vi "Stop All Processes.vi"() -> (0 "Stop Process":refnum<user-event>)   [LabVIEW 2011]
doc: "Creates a Stop Process user event."
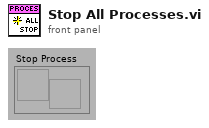
[diagram p1: front panel]
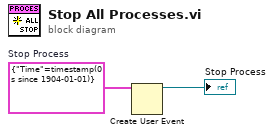
[diagram p0: block diagram]
diagram:
  w1 = cluster{"Time":timestamp} {"Time"=timestamp(0 s since 1904-01-01)}  # Stop Process
  n1 = Create User Event(user event datatype=w1) -> (user event=→"Stop Process":refnum<user-event>)  [unwired: 1 in, 1 out]
